vi "Setsource_mapped.vi"(8 "error in (no error)":errorcluster, 10 "Set_Val":T1, 11 "OneOfTemplate in":refnum<class "nixnet_grpc_ConnectTerminalsRequest_source_enum.lvclass">) -> (0 "error out":errorcluster, 3 "OneOfTemplate out":refnum<class "nixnet_grpc_ConnectTerminalsRequest_source_enum.lvclass">)   [LabVIEW 2019, in "xnet-grpc_client.lvlib" / "nixnet_grpc_ConnectTerminalsRequest_source_enum.lvclass"]
uses:
  nixnet_grpc_ConnectTerminalsRequest_source_enum.lvclass
  nixnet_grpc_TerminalName.ctl
  nixnet_grpc_ConnectTerminalsRequest_source_enum.lvclass/nixnet_grpc_ConnectTerminalsRequest_source_enum.ctl
  xnet-grpc_client.lvlib
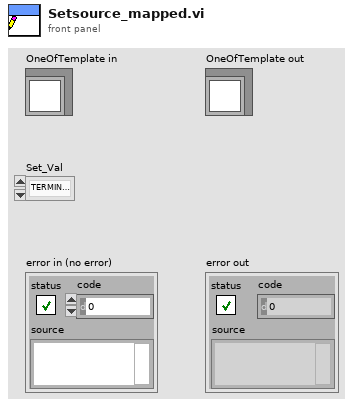
[diagram p1: front panel]
types:
  T1 = typedef "xnet-grpc_client.lvlib/nixnet_grpc_TerminalName.ctl" = enum32{"TERMINAL_NAME_UNSPECIFIED", "TERMINAL_NAME_PXI_TRIG_0", "TERMINAL_NAME_PXI_TRIG_1", "TERMINAL_NAME_PXI_TRIG_2", "TERMINAL_NAME_PXI_TRIG_3", "TERMINAL_NAME_PXI_TRIG_4", "TERMINAL_NAME_PXI_TRIG_5", "TERMINAL_NAME_PXI_TRIG_6", "TERMINAL_NAME_PXI_TRIG_7", "TERMINAL_NAME_FRONT_PANEL_0", "TERMINAL_NAME_FRONT_PANEL_1", "TERMINAL_NAME_PXI_STAR", "TERMINAL_NAME_PXI_CLK_10", "TERMINAL_NAME_10_MHZ_TIMEBASE", "TERMINAL_NAME_1_MHZ_TIMEBASE", "TERMINAL_NAME_MASTER_TIMEBASE", "TERMINAL_NAME_COMM_TRIGGER", "TERMINAL_NAME_START_TRIGGER", "TERMINAL_NAME_FLEX_RAY_START_CYCLE", "TERMINAL_NAME_FLEX_RAY_MACROTICK", "TERMINAL_NAME_LOG_TRIGGER", "TERMINAL_NAME_TIME_TRIGGER", "TERMINAL_NAME_NETWORK_TIME_PPS", "TERMINAL_NAME_NETWORK_TIME_1_MHZ"}
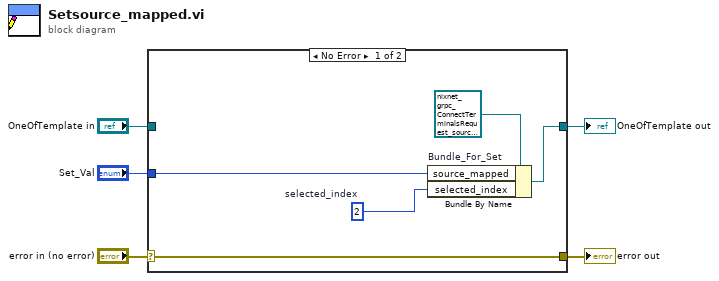
[diagram p0: block diagram]
diagram:
  n1 = case shown="No Error" "error in (no error)" {
    selector: "error in (no error)" -> [w10 w11]
    tunnel: [w10 w11] -> w4
    tunnel: [w9 w12] -> w2
    tunnel: "OneOfTemplate in" -> [_ w12]
    tunnel: "Set_Val" -> [w8 _]
    frame No Error {
      w7 = 2  # selected_index
      n2 = Bundle By Name "Bundle_For_Set"(cluster=refnum<class "nixnet_grpc_ConnectTerminalsRequest_source_enum.lvclass"> refnum ("OneOfTemplate in"), "source_mapped"=w8, "selected_index"=w7) -> (w9:refnum<class "nixnet_grpc_ConnectTerminalsRequest_source_enum.lvclass">)
    }
    frame Error {
    }
  }
  "error out" <- w4
  "OneOfTemplate out" <- w2
